vi "HFRR ADV v07.vi"() -> ()   [LabVIEW 2025] (continued)
                "state1" <- w4561
              }
              frame Enabled {
              }
            }
            n3602 = stacked-sequence {
              tunnel: w4478 -> [w4586 _ _]
              tunnel: [_ _ w4602] -> _
              frame #0 {
                (unwired) FALSE ("convert eol (F)")
                w4588 = enum16{"start", "end", "current"}."start" ("pos mode (0:2)")
                n3603 = local read "Path"() -> (w4582:path)
                n3604 = Path To String(path=w4582) -> (string=w4594:string)
                n3605 = Concatenate Strings(w4594, "\\", "Sensor File Name") -> (w4595:string)
                n3606 = local write "standard output 2"(" ") -> ()
                n3607 = String To Path(string=w4595) -> (path=w4585:path)
                n3608 = call <vilib>:"Open_Create_Replace File.vi"("advisory dialog? (display:T)"=FALSE, "function (open:0)"=T29."create or replace", "file path"=w4585) -> ("error out"=w4598:errorcluster, "refnum"=w4597:refnum<file>)  [unwired: 5 in, 2 out]
                n3609 = Set File Position(refnum=w4597, from (0:start)=w4588, error in=w4598) -> (refnum out=w4578:refnum<file>, error out=w4577:errorcluster)  [unwired: 1 in]
                n3610 = Write to Binary File(file (use dialog)=w4578, data=" ", error in=w4577, 5:FALSE ("prepend array or string size? (T)")) -> (refnum out=w4589:refnum<file>, error out=w4590:errorcluster)  [unwired: 2 in, 1 out]
                n3611 = Set File Position(offset (in bytes) (0)=w4588, refnum=w4589, error in=w4590) -> (refnum out=w4581:refnum<file>, error out=w4580:errorcluster)  [unwired: 1 in]
                n3612 = Write to Binary File(file (use dialog)=w4581, data=w4586, error in=w4580, 5:FALSE ("prepend array or string size? (T)")) -> (error out=w4584:errorcluster)  [unwired: 2 in, 2 out]
                n3613 = flat-sequence {
                  tunnel: w4585 -> [w4600]
                  tunnel: w4584 -> [_]
                  frame #0 {
                    n3614 = call <vilib>:"Read Characters From File.vi"("file path (dialog if empty)"=w4600) -> ("character string"=→"Sensor Health JSON string":string)  [unwired: 5 in, 3 out]
                  }
                }
                "SinglePoint  2" <- w4586
              }
              frame #1 {
              }
              frame #2 {
                (unwired) "\"Stored\": true" ("string")
                n3615 = call <vilib>:"System Exec.vi"("run minimized? (F)"=TRUE, "wait until completion? (T)"=TRUE, "working directory"=path "C:/LAB-IQ-NXT", "command line"="C:\\LAB-IQ-NXT\\JPostH.bat") -> ("standard error"=→"Respose From Server 2":string, "standard output"=w4605:string)  [unwired: 4 in, 2 out]
                "standard output 2" <- w4605
                n3616 = Match Pattern(string=w4605, regular expression="JSONH Check String") -> (match substring=w4603:string, offset past match=w4602:i32)  [unwired: 1 in, 2 out]
                n3617 = Equal?(x=w4603, y="JSONH Check String") -> (x = y?=→"Upload \nConfirmed 2":bool)
              }
            }
            n3618 = Divide(x=w4445, y=3600.0 ("f")) -> (x/y=w4438:dbl)
            n3619 = local read "run time"() -> (w4495:string[])
            n3620 = Round To Nearest(number=w4438) -> (nearest integer value=w4437:dbl)
            n3621 = Number To Decimal String(number=w4437) -> (decimal integer string=w4436:string)  [unwired: 1 in]
            n3622 = Index Array(array="Sensor Information", index (col) #1=0 ("disabled index (col)"), index (col) #2=1 ("index (col)"), index (col) #3=2 ("index (col)"), index (col) #4=3 ("index (col)")) -> (element #1=→"Sensor name":string[], element #2=→"model num":string[], element #3=→"run time":string[], element #4=→"state":string[])  [unwired: 4 in]
            n3623 = Insert Into Array(array=w4495, index=1, new element #1=w4436, new element #2=w4436, new element #3=w4436, new element #4=w4436, new element #5=w4436, new element #6=w4436) -> (w4460:string[])
            "run" <- w4460
            n3624 = local read "out"() -> (w4442:string[])
            n3625 = local read "Sensor Information"() -> (w4462:string[][])
            n3626 = Replace Array Subset(array=w4462, new element #1=w4460, index (col) #1=2 ("disabled index (col)"), new element #2=w4442, index (col) #2=3 ("index (col)")) -> (w4461:string[][])  [unwired: 2 in]
            n3627 = local write "Sensor Information"(w4461) -> ()
          }
        }
        n3628 = case shown="True" w4409 {
          frame False {
          }
          frame True {
            n3629 = Equal?(x="FLAG", y=0.0) -> (x = y?=w4426:bool)
            n3630 = case shown="False" w4426 {
              frame False {
                n3631 = Get Date/Time In Seconds() -> (seconds since 1Jan1904=w4432:timestamp)
                n3632 = local read "START 2"() -> (w4430:dbl)
                n3633 = To Double Precision Float(number=w4432) -> (double precision float=w4431:dbl)
                n3634 = Subtract(x=w4431, y=w4430) -> (x-y=→"SENSOR TIME  2":dbl)
              }
              frame True {
                n3635 = Get Date/Time In Seconds() -> (seconds since 1Jan1904=w4434:timestamp)
                n3636 = To Double Precision Float(number=w4434) -> (double precision float=→"START 2":dbl)
                n3637 = local write "FLAG"(100.0 ("FLAG")) -> ()
              }
            }
          }
        }
        n3638 = disable-structure shown="Disabled" {
          disable-tunnel: w4412 -> [w4421 _]
          disable-tunnel: [w4420 _] -> w4411
          frame Disabled {
            n3639 = local read "Json St Flg"() -> (w4419:bool)
            n3640 = case shown="True" w4419 {
              tunnel: w4421 -> [w4422 w4424]
              tunnel: [w4422 w4423] -> w4420
              frame False {
              }
              frame True {
                n3641 = Increment(x=w4424) -> (x+1=w4423:dbl)
                "T cycle" <- w4423
                n3642 = local write "Json St Flg"(FALSE ("Json St Flg")) -> ()
              }
            }
          }
          frame Enabled {
          }
        }
        n3643 = local read "Quit"() -> (w4406:bool)
      }
    }
    frame Enabled {
    }
  }
  n3644 = stacked-sequence {
    tunnel: [w4804] -> w38
    frame #0 {
      w4804 = FALSE ("Upload \nConfirmed")
      n3645 = local write "Upload \nConfirmed"(w4804) -> ()
      n3646 = local write "St Str"("") -> ()
    }
  }
  n3647 = disable-structure shown="Disabled" {
    disable-tunnel: w38 -> [w4805 _]
    frame Disabled {
      n3648 = case shown="True" {
        selector: _ -> [_ _]
        tunnel: w4805 -> [_ w4806]
        frame False {
        }
        frame True {
          n3649 = while {
            tunnel: [w4812] -> _
            tunnel: w4806 -> [_]
            i -> [w4812]
            stop <- w4807 stop-if-true
            n3650 = local read "Json End Flg"() -> (w4811:bool)
            n3651 = Wait (ms)(milliseconds to wait=u32 20 ("Refresh Rate (ms)")) -> ()  [unwired: 1 out]
            n3652 = local read "refresh flag"() -> (w4808:bool)
            n3653 = local read "RUN"() -> (w4809:bool)
            n3654 = And(x=w4809, y=w4808) -> (x .and. y?=w4810:bool)
            n3655 = Or(x=w4810, y=w4811) -> (x .or. y?=w4813:bool)
            "AR Led" <- w4813
            n3656 = case shown="True" w4813 {
              frame False {
              }
              frame True {
                w4830 = "\",\""
                n3657 = local read "UUID"() -> (w4828:string)
                n3658 = local write "refresh flag"(FALSE ("refresh flag")) -> ()
                n3659 = local read "time"() -> (w4817:dbl)
                n3660 = Multiply(x=w4817, y=60.0) -> (x*y=w4816:dbl)
                n3661 = Concatenate Strings("UUID\" : \"", w4828, "\"}") -> (w4831:string)
                n3662 = Number To Fractional String(number=w4816, width (-)=i16 10, precision (6)=i16 4) -> (F-format string=w4845:string)  [unwired: 1 in]
                n3663 = Concatenate Strings("{", "\"Time\":\"", w4845, w4830) -> (w4840:string)
                n3664 = stacked-sequence {
                  tunnel: w4830 -> [w4893 w4901 w4908 w4916 w4924 w4933 w4940]
                  tunnel: [w4894 _ _ _ _ _ _] -> w4844
                  tunnel: [_ w4902 _ _ _ _ _] -> w4843
                  tunnel: [_ _ w4909 _ _ _ _] -> w4842
                  tunnel: [_ _ _ w4918 _ _ _] -> w4841
                  tunnel: w4831 -> [_ _ _ _ _ _ w4951]
                  tunnel: [_ _ _ _ _ _ w4950] -> w4827
                  tunnel: [_ _ _ _ _ w4930 _] -> w4826
                  tunnel: [_ _ _ _ w4923 _ _] -> w4825
                  frame #0 {
                    n3665 = local read "NORMAL LOAD"() -> (w4892:dbl)
                    n3666 = Number To Fractional String(number=w4892, width (-)=i16 10, precision (6)=i16 4) -> (F-format string=w4895:string)  [unwired: 1 in]
                    n3667 = Concatenate Strings("NormalLoad\":\"", w4895, w4893) -> (w4894:string)
                  }
                  frame #1 {
                    n3668 = local read "Temp"() -> (w4900:dbl)
                    n3669 = Number To Fractional String(number=w4900, width (-)=i16 10, precision (6)=i16 4) -> (F-format string=w4903:string)  [unwired: 1 in]
                    n3670 = Concatenate Strings("Temperature\":\"", w4903, w4901) -> (w4902:string)
                  }
                  frame #2 {
                    n3671 = local read "cof"() -> (w4906:dbl)
                    n3672 = Number To Fractional String(number=w4906, width (-)=i16 10, precision (6)=i16 4) -> (F-format string=w4910:string)  [unwired: 1 in]
                    n3673 = Concatenate Strings("FrictionalForce\":\"", w4910, w4908) -> (w4909:string)
                  }
                  frame #3 {
                    n3674 = local read "Set Hz"() -> (w4914:dbl)
                    n3675 = Multiply(x=w4914, y=60.0) -> (x*y=w4913:dbl)
                    n3676 = Number To Fractional String(number=w4913, width (-)=i16 10, precision (6)=i16 4) -> (F-format string=w4919:string)  [unwired: 1 in]
                    n3677 = Concatenate Strings("Speed\":\"", w4919, w4916) -> (w4918:string)
                  }
                  frame #4 {
                    n3678 = local read item#-1() -> (w4922)
                    n3679 = Number To Fractional String(number=w4922, width (-)=i16 10, precision (6)=i16 4) -> (F-format string=w4926:string)  [unwired: 1 in]
                    n3680 = Concatenate Strings("LinearDeformation\":\"", w4926, w4924) -> (w4923:string)
                  }
                  frame #5 {
                    n3681 = local read "AIR TEMP"() -> (w4929:dbl)
                    n3682 = local read "Json St Flg"() -> (w4931:bool)
                    n3683 = local read "Json End Flg"() -> (w4932:bool)
                    n3684 = Number To Fractional String(number=w4929, width (-)=i16 10, precision (6)=i16 4) -> (F-format string=w4935:string)  [unwired: 1 in]
                    n3685 = Concatenate Strings("Vibration\":\"", w4935, w4933) -> (w4930:string)
                    n3686 = And(x=w4931, y=w4932) -> ()  [unwired: 1 out]
                  }
                  frame #6 {
                    n3687 = local read "Json End Flg"() -> (w4939:bool)
                    n3688 = Get Date/Time In Seconds() -> (seconds since 1Jan1904=w4947:timestamp)
                    n3689 = local read "Json St Flg"() -> (w4938:bool)
                    n3690 = To Double Precision Float(number=w4947) -> (double precision float=w4946:dbl)
                    n3691 = Subtract(x=w4946, y=2082844800.0) -> (x-y=w4944:dbl)
                    n3692 = Number To Fractional String(number=w4944, width (-)=i16 12, precision (6)=i16 0) -> (F-format string=w4941:string)  [unwired: 1 in]
                    n3693 = case shown="True" w4939 {
                      tunnel: ["" w4954] -> w4948
                      tunnel: w4941 -> [_ w4955]
                      tunnel: w4940 -> [_ w4953]
                      frame False {
                      }
                      frame True {
                        n3694 = local write "Json End Flg"(FALSE ("Json St Flg")) -> ()
                        n3695 = Concatenate Strings("End\": \"", w4955, w4953) -> (w4954:string)
                      }
                    }
                    n3696 = case shown="True" w4938 {
                      tunnel: [w4958 w4961] -> w4949
                      tunnel: w4941 -> [_ w4962]
                      tunnel: w4940 -> [_ w4959]
                      frame False {
                        n3697 = local read "St Str"() -> (w4958:string)
                      }
                      frame True {
                        n3698 = Concatenate Strings("Start\":\"", w4962, w4959) -> (w4961:string)
                        "St Str" <- w4961
                        n3699 = local write "Json St Flg"(FALSE ("Json St Flg")) -> ()
                      }
                    }
                    n3700 = Concatenate Strings(w4949, w4948, w4951) -> (w4950:string)
                  }
                }
                n3701 = local read "FILE"() -> (w4819:string)
                n3702 = Concatenate Strings("\",\"DatasetTitle\":\"" ("string"), w4819) -> (w4821:string)
                n3703 = Concatenate Strings("\",\"OperatorID\":\"" ("string"), "Operator ID") -> (w4822:string)
                n3704 = Concatenate Strings("\",\"ModelNumber\":\"" ("string"), "Model No") -> (w4850:string)
                n3705 = Concatenate Strings("\",\"SerialNumber\":\"" ("string"), "Serial No") -> (w4851:string)
                n3706 = Concatenate Strings(w4851, w4850) -> (w4833:string)
                n3707 = Concatenate Strings("{\"SecretKey\":\"", "Secret Key", w4833, w4822, w4821, "\",\"Samples\":[") -> (w4838:string)
                n3708 = Concatenate Strings(w4840, w4844, w4843, w4842, w4841, w4825, w4826, w4827) -> (w4839:string)
                n3709 = Concatenate Strings(w4838, w4839, "]}") -> (w4837:string)
                n3710 = stacked-sequence {
                  tunnel: w4837 -> [w4866 _ _]
                  tunnel: [_ _ w4883] -> _
                  frame #0 {
                    (unwired) FALSE ("convert eol (F)")
                    w4868 = enum16{"start", "end", "current"}."start" ("pos mode (0:2)")
                    n3711 = Path To String(path="Path") -> (string=w4874:string)
                    n3712 = Concatenate Strings(w4874, "\\", "Data File Name") -> (w4876:string)
                    n3713 = local write "standard output"(" ") -> ()
                    n3714 = String To Path(string=w4876) -> (path=w4865:path)
                    n3715 = call <vilib>:"Open_Create_Replace File.vi"("advisory dialog? (display:T)"=FALSE, "function (open:0)"=T29."create or replace", "file path"=w4865) -> ("error out"=w4879:errorcluster, "refnum"=w4878:refnum<file>)  [unwired: 5 in, 2 out]
                    n3716 = Set File Position(refnum=w4878, from (0:start)=w4868, error in=w4879) -> (refnum out=w4859:refnum<file>, error out=w4858:errorcluster)  [unwired: 1 in]
                    n3717 = Write to Binary File(file (use dialog)=w4859, data=" ", error in=w4858, 5:FALSE ("prepend array or string size? (T)")) -> (refnum out=w4869:refnum<file>, error out=w4870:errorcluster)  [unwired: 2 in, 1 out]
                    n3718 = Set File Position(offset (in bytes) (0)=w4868, refnum=w4869, error in=w4870) -> (refnum out=w4862:refnum<file>, error out=w4861:errorcluster)  [unwired: 1 in]
                    n3719 = Write to Binary File(file (use dialog)=w4862, data=w4866, error in=w4861, 5:FALSE ("prepend array or string size? (T)")) -> (error out=w4864:errorcluster)  [unwired: 2 in, 2 out]
                    n3720 = flat-sequence {
                      tunnel: w4865 -> [w4881]
                      tunnel: w4864 -> [_]
                      frame #0 {
                        n3721 = call <vilib>:"Read Characters From File.vi"("file path (dialog if empty)"=w4881) -> ("character string"=→"JSON string":string)  [unwired: 5 in, 3 out]
                      }
                    }
                    "SinglePoint" <- w4866
                  }
                  frame #1 {
                  }
                  frame #2 {
                    (unwired) "\"Stored\": true" ("string")
                    n3722 = call <vilib>:"System Exec.vi"("run minimized? (F)"=TRUE, "wait until completion? (T)"=TRUE, "working directory"=path "C:/LAB-IQ-NXT", "command line"="C:\\LAB-IQ-NXT\\JPost.bat") -> ("standard error"=→"Respose From Server":string, "standard output"=w4886:string)  [unwired: 4 in, 2 out]
                    "standard output" <- w4886
                    n3723 = Match Pattern(string=w4886, regular expression="JSON Check String") -> (match substring=w4884:string, offset past match=w4883:i32)  [unwired: 1 in, 2 out]
                    n3724 = Equal?(x=w4884, y="JSON Check String") -> (x = y?=→"Upload \nConfirmed":bool)
                  }
                }
              }
            }
            n3725 = local read "Quit"() -> (w4807:bool)
          }
        }
      }
    }
    frame Enabled {
    }
  }
  n3726 = disable-structure shown="Disabled" {
    disable-tunnel: _ -> [w4969 _]
    frame Disabled {
      n3727 = while {
        shift-right: [w4977] -> w4965
        shift-left: _ -> [w4978]
        shift-right: [w4975] -> w4966
        shift-left: errorcluster {"status"=TRUE, "code"=0, "source"="Init"} ("error out") -> [w4976]
        shift-right: [w4973] -> _
        shift-left: "" -> [w4974]
        tunnel: [w4971] -> _
        tunnel: w4969 -> [_]
        i -> [w4971]
        stop <- w4970 stop-if-true
        n3728 = flat-sequence {
          tunnel: [w4979] -> w4972
          frame #0 {
            n3729 = Wait (ms)(milliseconds to wait=10.0 ("Delay")) -> (millisecond timer value=w4979:u32)
          }
        }
        n3730 = case shown="No Error" w4976 {
          selector: w4976 -> [w5009 w5128]
          tunnel: [w4992 w5130] -> w4977
          tunnel: [w4991 w5129] -> w4975
          tunnel: w4978 -> [w5010 w5122]
          tunnel: w4974 -> [w4990 w5121]
          tunnel: [w4989 w5121] -> w4973
          tunnel: w4972 -> [_ _]
          frame No Error {
            n3731 = Concatenate Strings("\r", "\n") -> (w5001:string)  [unwired: 1 in]
            n3732 = case shown="True" w5002 {
              tunnel: w5010 -> [w5034 w5041]
              tunnel: w5009 -> [w5033 w5040]
              tunnel: [w5034 w5039] -> w5008
              tunnel: [w5033 w5038] -> w4988
              tunnel: w5001 -> [_ w5037]
              frame False {
              }
              frame True {
                n3733 = VISA Write(VISA resource name=w5041, write buffer=w5037, error in (no error)=w5040) -> (VISA resource name out=w5039:refnum<visa-resource-name>, error out=w5038:errorcluster)  [unwired: 1 out]
                n3734 = local write "Read String"("") -> ()
                n3735 = local write item#-1(FALSE) -> ()
              }
            }
            n3736 = property class="Instr"(reference=w5008, error in=w4988) -> (reference out=w5007:refnum<visa-resource-name>, error out=w5006:errorcluster, "Serial Settings:Number of Bytes at Serial Port"=w5005:u32)
            n3737 = Greater?(x=w5005, y=u32 100) -> (0:w5003:bool)
            n3738 = case shown="True" w5003 {
              tunnel: w5007 -> [w5044 w5068]
              tunnel: w5006 -> [w5043 w5067]
              tunnel: w5005 -> [_ w5066]
              tunnel: [w5044 w5065] -> w4994
              tunnel: [w5043 w5064] -> w4993
              tunnel: w4990 -> [w5042 w5063]
              tunnel: [w5042 ""] -> w4989
              frame False {
              }
              frame True {
                w5053 = u32 6 ("y")
                # "Page 84 of \nmanual"
                n3739 = VISA Read(VISA resource name=w5068, byte count=w5066, error in (no error)=w5067) -> (VISA resource name out=w5065:refnum<visa-resource-name>, read buffer=w5061:string, error out=w5064:errorcluster)  [unwired: 1 out]
                n3740 = while {
                  tunnel: w5061 -> [w5117]
                  tunnel: [w5113] -> w5055 mode=indexing
                  tunnel: [w5107] -> w5059 mode=indexing
                  tunnel: [w5105] -> _
                  i -> [w5105]
                  stop <- w5110 stop-if-true
                  n3741 = String Subset(string=w5117, offset (0)=w5105) -> (substring=w5112:string)  [unwired: 1 in]
                  n3742 = String To Byte Array(string=w5112) -> (unsigned byte array=w5116:u8[])
                  n3743 = String Length(string=w5112) -> (length=w5111:i32)
                  n3744 = Index Array(array=w5116) -> (element=w5115:u8)  [unwired: 1 in]
                  n3745 = Equal To 0?(x=w5111) -> (x = 0?=w5110:bool)
                  n3746 = Number To Boolean Array(number=w5115) -> (Boolean array=w5109:bool[])
                  n3747 = Reverse 1D Array(array=w5109) -> (reversed array=w5108:bool[])
                  n3748 = And(x=w5109, y=bool[] [FALSE, FALSE, FALSE, FALSE, FALSE, FALSE, TRUE, TRUE] ("Boolean array")) -> (x .and. y?=w5113:bool[])
                  n3749 = And(x=w5108, y=bool[] [FALSE, FALSE, TRUE, TRUE, TRUE, TRUE, TRUE, TRUE] ("Boolean array")) -> (x .and. y?=w5107:bool[])
                }
                n3750 = Concatenate Strings(w5063, w5061) -> (→"Read String":string)
                n3751 = while {
                  tunnel: w5055 -> [w5104] mode=indexing
                  tunnel: [w5100] -> w5058
                  i -> [w5100]
                  stop <- w5101 stop-if-true
                  n3752 = Search 1D Array(1D array=w5104, element=TRUE) -> (index of element=w5102:i32)  [unwired: 1 in]
                  n3753 = Less Than 0?(x=w5102) -> (x < 0?=w5101:bool)
                }
                n3754 = Delete From Array(array=w5059, length=w5058, index (row)=0) -> (array with subset deleted=w5054:bool[][])  [unwired: 1 in, 1 out]
                n3755 = Array Size(array=w5054) -> (size(s)=w5056:i32[])
                n3756 = Index Array(array=w5056) -> (element=w5048:i32)  [unwired: 1 in]
                n3757 = Greater?(x=w5048, y=w5053) -> (0:w5051:bool)
                n3758 = Subtract(x=w5048, y=w5053) -> (x-y=w5052:u32)
                n3759 = Select(t=w5052, s=w5051, f=u32 0) -> (s? t:f=w5049:u32)
                n3760 = while {
                  tunnel: w5054 -> [w5087]
                  tunnel: [w5089] -> w5047 mode=indexing
                  tunnel: w5049 -> [w5071]
                  i -> [w5088]
                  stop <- w5086 stop-if-true
                  w5078 = 6 ("index")
                  w5077 = 2 ("length")
                  # "Page 65 of \nmanual"
                  n3761 = Multiply(x=u32 3 ("y"), y=w5088) -> (x*y=w5085:u32)
                  n3762 = Divide(x=u32 102 ("y"), y=u32 65520) -> (x/y=w5095:dbl)
                  n3763 = Greater Or Equal?(x=w5085, y=w5071) -> (x >= y?=w5086:bool)
                  n3764 = Index Array(array=w5087, index (row) #1=w5085) -> (element #1=w5083:bool[], element #2=w5082:bool[], element #3=w5081:bool[])  [unwired: 5 in]
                  n3765 = Reverse 1D Array(array=w5083) -> (reversed array=w5076:bool[])
                  n3766 = Reverse 1D Array(array=w5081) -> (reversed array=w5079:bool[])
                  n3767 = Reverse 1D Array(array=w5082) -> (reversed array=w5080:bool[])
                  n3768 = Delete From Array(array=w5080, length=w5077, index=w5078) -> (array with subset deleted=w5073:bool[])  [unwired: 1 out]
                  n3769 = Delete From Array(array=w5076, length=w5077, index=w5078) -> (array with subset deleted=w5072:bool[])  [unwired: 1 out]
                  n3770 = Delete From Array(array=w5079, length=w5077, index=w5078) -> (array with subset deleted=w5074:bool[])  [unwired: 1 out]
                  n3771 = Insert Into Array(array=bool[] [] ("Boolean array"), new element #1=w5072, new element #2=w5073, new element #3=w5074) -> (w5075:bool[])  [unwired: 1 in]
                  n3772 = Boolean Array To Number(Boolean array=w5075) -> (number=w5084:u32)
                  n3773 = Multiply(x=w5095, y=w5084) -> (x*y=w5094:dbl)
                  n3774 = Decrement(x=w5094) -> (x-1=w5093:dbl)
                  n3775 = Divide(x=w5093, y=u32 100) -> (x/y=w5091:dbl)
                  n3776 = Multiply(x=w5091, y=u32 10) -> (x*y=w5089:dbl)
                }
                n3777 = Delete From Array(array=w5047) -> (array with subset deleted=w5046:dbl[])  [unwired: 2 in, 1 out]
                "Waveform Graph 5" <- w5046
                "Waveform Chart 3" <- w5046
                n3778 = call-poly <vilib>:"Mean.vi"("X"=w5046) -> ("mean"=w5045:dbl)  [unwired: 1 out]
                n3779 = case shown="True" {
                  selector: _ -> [_ _]
                  tunnel: w5045 -> [_ w5070]
                  frame False {
                  }
                  frame True {
                    n3780 = local write item#-1(FALSE ("Zero 4")) -> ()
                    "z_measure" <- w5070
                  }
                }
              }
            }
            n3781 = local read item#-1() -> (w4985)
            n3782 = local read item#-1() -> (w4986)
            n3783 = local read item#-1() -> (w4984)
            n3784 = local read item#-1() -> (w4983)
            n3785 = case shown="True" w4981 {
              tunnel: w4985 -> [_ w5013]
              tunnel: w4986 -> [_ w5012]
              frame False {
              }
              frame True {
                n3786 = Build Array(w5013, w5012) -> (w5011:void[])
                n3787 = local read item#-1() -> (w5016)
                n3788 = Build Array (concatenate)(w5016, w5011) -> (w5014:void[])
                n3789 = local write item#-1(w5014) -> ()
                n3790 = local write item#-1(FALSE ("Boolean 8")) -> ()
              }
            }
            n3791 = call "Build XY Graph"("Enable"=w4983, "Reset"=w4984, "Y Input"=w4986, "X Input"=w4985) -> ("XY Graph"=w4982:cluster{"Y":dbl[], "Y":dbl[]}[])  [unwired: 6 in, 1 out]
            n3792 = case shown="True" {
              selector: _ -> [_ _]
              frame False {
              }
              frame True {
                n3793 = local read item#-1() -> (w5017)
                n3794 = Index Array(array=w5017, index (col) #1=0 ("disabled index (col)"), index (col) #2=1 ("index (col)")) -> (element #1=w5019, element #2=w5018)  [unwired: 2 in]
                n3795 = call <vilib>:"Linear Fit.vi"("Y"=w5019, "X"=w5018) -> ()  [unwired: 9 in, 5 out]
                n3796 = local write item#-1(FALSE ("Boolean 9")) -> ()
              }
            }
            n3797 = case shown="True" {
              selector: _ -> [_ _]
              frame False {
              }
              frame True {
                n3798 = local write item#-1(dbl[][] [] ("Captured Values")) -> ()
                n3799 = local write item#-1(FALSE ("Boolean 7")) -> ()
              }
            }
            n3800 = Concatenate Strings("\r", "\n") -> (w4996:string, w4995:string)
            n3801 = case shown="True" w4987 {
              tunnel: w4994 -> [w5026 w5032]
              tunnel: w4993 -> [w5025 w5031]
              tunnel: [w5026 w5030] -> w4992
              tunnel: [w5025 w5029] -> w4991
              tunnel: w4996 -> [_ w5028]
              frame False {
              }
              frame True {
                n3802 = VISA Write(VISA resource name=w5032, write buffer=w5028, error in (no error)=w5031) -> (VISA resource name out=w5030:refnum<visa-resource-name>, error out=w5029:errorcluster)  [unwired: 1 out]
                n3803 = local write item#-1(FALSE ("WRITE")) -> ()
              }
            }
          }
          frame Error {
            w5120 = u16 10 items=["1.0"=10, "1.5"=15, "2.0"=20] ("stop bits (10: 1 bit)")
            n3804 = Wait (ms)(milliseconds to wait=u32 20) -> ()  [unwired: 1 out]
            n3805 = VISA Close(VISA resource name=w5122, error in (no error)=w5128) -> (error out=w5127:errorcluster)
            n3806 = call <vilib>:"Clear Errors.vi"("error in (no error)"=w5127) -> ("error out"=w5126:errorcluster)  [unwired: 5 in, 1 out]
            n3807 = call-poly "VISA Configure Serial Port"("timeout (10sec)"=u32 200, "Enable Termination\nChar (T)"=TRUE ("Enable Termination\nChar (T)"), "baud rate (9600)"=u32 921600, "error in (no error)"=w5126, "stop bits (10: 1 bit)"=w5120) -> ("VISA resource name"=w5118:refnum<visa-resource-name>, "VISA resource name out"=w5130:refnum<visa-resource-name>, "error out"=w5129:errorcluster)  [unwired: 8 in]
          }
        }
        n3808 = local read "Quit"() -> (w4970:bool)
      }
      n3809 = VISA Close(VISA resource name=w4965, error in (no error)=w4966) -> (error out=w4964:errorcluster)
      n3810 = call <vilib>:"Clear Errors.vi"("error in (no error)"=w4964) -> ()  [unwired: 5 in, 2 out]
    }
    frame Enabled {
    }
  }
  n3811 = disable-structure shown="Disabled" {
    disable-tunnel: _ -> [w5135 _]
    frame Disabled {
      n3812 = while {
        tunnel: [w5142] -> _
        shift-right: [w5139] -> w5132
        shift-left: _ -> [w5141]
        shift-right: [w5140] -> w5133
        shift-left: errorcluster {"status"=TRUE, "code"=0, "source"="Init"} ("error out") -> [w5138]
        tunnel: w5135 -> [_]
        i -> [w5142]
        stop <- w5136 stop-if-true
        n3813 = flat-sequence {
          tunnel: w5138 -> [w5233]
          tunnel: [w5233] -> w5137
          frame #0 {
            n3814 = Wait (ms)(milliseconds to wait=u32 50) -> ()  [unwired: 1 out]
          }
        }
        n3815 = case shown="No Error" w5137 {
          selector: w5137 -> [w5183 w5226]
          tunnel: w5141 -> [w5182 w5225]
          tunnel: [w5149 w5216] -> w5140
          tunnel: [w5150 w5224] -> w5139
          frame No Error {
            w5176 = T30 {"Mode"=enum."RTU", "Slave Address"=1} ("Serial Parameters")
            n3816 = call-poly <vilib>:"MB Serial Master Query (poly).vi"("VISA resource name"=w5182, "Starting Address"=i16 1000, "Quantity"=u16 1, "Timeout"=u32 1000, "error in"=w5183, "Serial Parameters"=w5176) -> ("VISA resource name out"=w5177:refnum<visa-resource-name>, "Input Registers"=w5179:u16[], "error out"=w5175:errorcluster)  [unwired: 10 in, 1 out]
            n3817 = Random Number (0-1)() -> (number: 0 to 1=w5164:dbl)
            n3818 = Index Array(array=w5179, index=0) -> (element=w5174:u16)
            n3819 = Subtract(x=w5164, y=0.5) -> (x-y=w5163:dbl)
            n3820 = Divide(x=w5174, y=10 ("index")) -> (x/y=w5168:dbl)
            n3821 = Multiply(x=w5163, y=0.5) -> (x*y=w5162:dbl)
            n3822 = Add(x=w5168, y=w5162) -> (x+y=w5167:dbl)
            n3823 = local read "Amb temp"() -> (w5151:dbl)
            n3824 = Multiply(x=w5167, y=0.2) -> (x*y=w5171:dbl)
            n3825 = Multiply(x=w5151, y=0.8) -> (x*y=w5169:dbl)
            n3826 = Add(x=w5171, y=w5169) -> (x+y=w5152:dbl)
            n3827 = local read "set temp old"() -> (w5146:dbl)
            n3828 = local write "Amb temp"(w5152) -> ()
            n3829 = Select(t="SetTemp 2", s="Heater", f=100.0) -> (s? t:f=w5147:dbl)
            n3830 = Not Equal?(x=w5147, y=w5146) -> (x != y?=w5145:bool)
            n3831 = case shown="True" w5145 {
              tunnel: w5177 -> [w5211 w5213]
              tunnel: [w5210 w5213] -> w5157
              tunnel: w5175 -> [w5209 w5212]
              tunnel: [w5208 w5212] -> w5155
              tunnel: w5147 -> [w5203 _]
              tunnel: w5176 -> [w5205 w5214]
              tunnel: [w5205 w5214] -> w5158
              frame True {
                n3832 = Multiply(x=w5203, y=10 ("index")) -> (x*y=w5202:dbl)
                n3833 = call-poly <vilib>:"MB Serial Master Query (poly).vi"("VISA resource name"=w5211, "Address"=u16 0, "Holding Register"=w5202, "Timeout"=u32 1000, "error in"=w5209, "Serial Parameters"=w5205) -> ("VISA resource name out"=w5210:refnum<visa-resource-name>, "error out"=w5208:errorcluster)  [unwired: 11 in, 1 out]
                "set temp old" <- w5203
              }
              frame False {
              }
            }
            n3834 = flat-sequence {
              tunnel: [w5184] -> _
              tunnel: [w5184] -> w5154
              tunnel: w5155 -> [w5184]
              frame #0 {
                n3835 = Wait (ms)(milliseconds to wait=u32 100) -> ()  [unwired: 1 out]
              }
            }
            n3836 = call "Elapsed Time12"("Time Target (s)"=2.0, "Auto Reset"=TRUE) -> ("Time has Elapsed"=w5159:bool)  [unwired: 10 in, 7 out]
            n3837 = case shown="True" w5159 {
              tunnel: w5158 -> [w5188 w5201]
              tunnel: [w5188 w5201] -> _
              tunnel: [w5187 w5199] -> w5150
              tunnel: w5157 -> [w5187 w5200]
              tunnel: [w5186 w5197] -> w5149
              tunnel: w5154 -> [w5186 w5198]
              frame False {
              }
              frame True {
                n3838 = call-poly <vilib>:"MB Serial Master Query (poly).vi"("VISA resource name"=w5200, "Starting Address"=i16 1003 ("Addr"), "Quantity"=u16 1, "Timeout"=u32 1000, "error in"=w5198, "Serial Parameters"=w5201) -> ("VISA resource name out"=w5199:refnum<visa-resource-name>, "Input Registers"=w5194:u16[], "error out"=w5197:errorcluster)  [unwired: 10 in, 1 out]
                n3839 = Index Array(array=w5194, index=0) -> (element=w5193:u16)
                n3840 = Divide(x=w5193, y=u16 10) -> (x/y=w5189:dbl)
                n3841 = local write "set temp old"(w5189) -> ()
                n3842 = local write "SetTemp"(w5189) -> ()
              }
            }
            "Error Code" <- w5149
            n3843 = Unbundle(w5149) -> ("status"=→"TK4 status":bool)  [unwired: 2 out]
            "SetTemp" <- "SetTemp 2"
          }
          frame Error {
            w5228 = u16 0 items=["None", "Odd", "Even", "Mark", "Space"] ("Parity")
            w5229 = u16 0 items=["None", "XON/XOFF", "RTS/CTS", "XON/XOFF & RTS/CTS", "DTR/DSR", "XON/XOFF & DTR/DSR"] ("Flow Control")
            n3844 = VISA Clear(VISA resource name=w5225, error in (no error)=w5226) -> (VISA resource name out=w5219:refnum<visa-resource-name>, error out=w5217:errorcluster)
            n3845 = VISA Close(VISA resource name=w5219, error in (no error)=w5217) -> (error out=w5218:errorcluster)
            n3846 = call <vilib>:"Clear Errors.vi"("error in (no error)"=w5218) -> ("error out"=w5227:errorcluster)  [unwired: 5 in, 1 out]
            n3847 = Unbundle By Name(T30 {"Mode"=enum."RTU", "Slave Address"=1} ("input cluster")) -> ("Mode"=w5230:enum16{"RTU", "ASCII"})
            n3848 = call <vilib>:"MB Serial Init.vi"("Timeout"=u32 100, "Flow Control"=w5229, "Mode"=w5230, "error in (no error)"=w5227, "Parity"=w5228, "Baud Rate"=u32 9600, "VISA resource name"="Lubrication System COM Port :") -> ("error out"=w5216:errorcluster, "VISA resource name out"=w5224:refnum<visa-resource-name>)  [unwired: 3 in]
            n3849 = local write "set temp old"(0.0 ("set temp old")) -> ()
            n3850 = Unbundle(w5216) -> ("status"=w5215:bool)  [unwired: 2 out]
            n3851 = case shown="True" w5215 {
              selector: w5215 -> [_ w5232]
              frame False {
              }
              frame True {
                n3852 = local write "TK4 status"(w5232) -> ()
              }
            }
          }
        }
        n3853 = local read "Quit"() -> (w5136:bool)
      }
      n3854 = VISA Close(VISA resource name=w5132, error in (no error)=w5133) -> (error out=w5131:errorcluster)
      n3855 = call <vilib>:"Clear Errors.vi"("error in (no error)"=w5131) -> ()  [unwired: 5 in, 2 out]
    }
    frame Enabled {
    }
  }
